vi "Generated Code.vi"   [LabVIEW 2014]
uses:
  SPIBus0/IO Node Logic Template_SPIBus0.lvlib
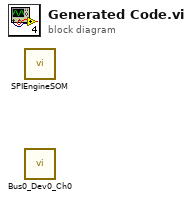
[diagram p0: block diagram]
diagram:
  n1 = call "SPIEngineSOM.vi"() -> ()  [unwired: 12 in]
  n2 = call "Bus0_Dev0_Ch0.vi"() -> ()  [unwired: 15 in, 1 out]
